vi "Pulsewidth.vi"(7 "Current Tick count":u32, 8 "Previous Updated Pulsewidth in":u32, 9 "Current Pulse Width In":u32, 10 "Prev. Echo Line State":bool, 11 "Echo Line State":bool) -> (0 "Updated Pulsewidth out":u32, 1 "Current Pulsewidth out":u32)   [LabVIEW 2014]
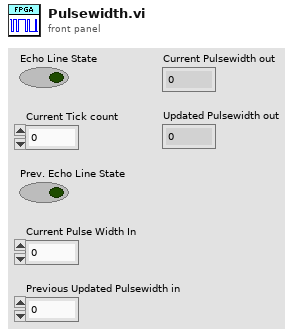
[diagram p1: front panel]
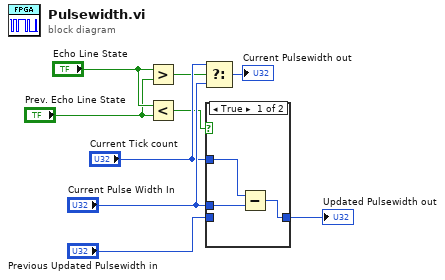
[diagram p0: block diagram]
diagram:
  n1 = Greater?(x="Echo Line State", y="Prev. Echo Line State") -> (0:w1:bool)
  n2 = Less?(x="Echo Line State", y="Prev. Echo Line State") -> (x < y?=w2:bool)
  n3 = Select(t="Current Tick count", s=w1, f="Current Pulse Width In") -> (s? t:f=→"Current Pulsewidth out":u32)
  n4 = case shown="True" w2 {
    tunnel: "Previous Updated Pulsewidth in" -> [_ w13]
    tunnel: "Current Tick count" -> [w10 _]
    tunnel: "Current Pulse Width In" -> [w11 _]
    tunnel: [w12 w13] -> w9
    frame True {
      n5 = Subtract(x=w10, y=w11) -> (x-y=w12:u32)
    }
    frame False {
    }
  }
  "Updated Pulsewidth out" <- w9
